vi "PAX_Read.vi"(8 "error in (no error)":errorcluster {"code" format="%.0x"}, 11 "VISA in":refnum<visa-resource-name> caption="instrument handle") -> (0 "error out":errorcluster {"code" format="%.0x"}, 1 "DOP":dbl, 2 "Azimuth deg":dbl, 3 "VISAout":refnum<visa-resource-name> caption="instrument handle out", 4 "s1":dbl, 5 "Ellipticity deg":dbl caption="Ellipticity rad", 6 "s3":dbl, 7 "s2":dbl)   [LabVIEW 2018]
panel:
  out "Total Power":dbl
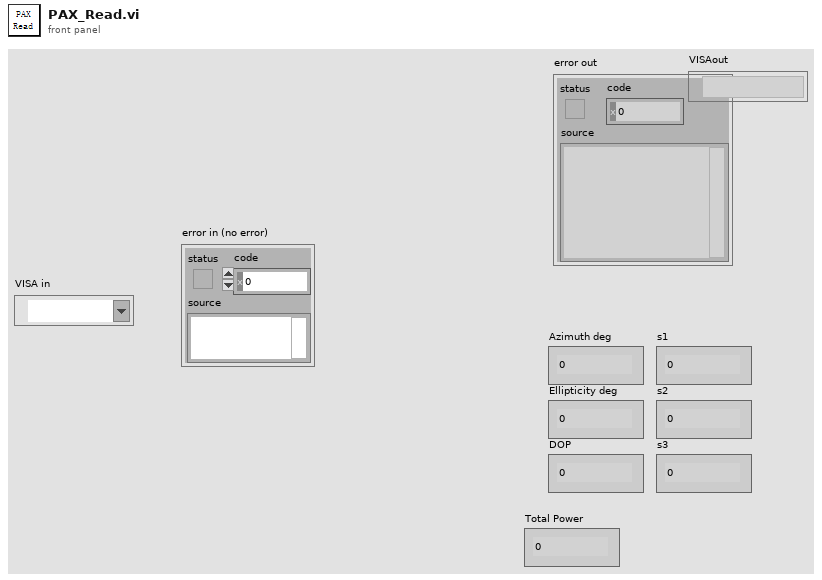
[diagram p1: front panel]
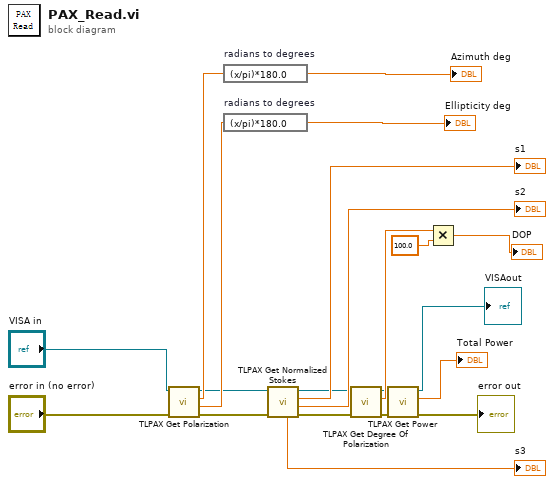
[diagram p0: block diagram]
diagram:
  n1 = call <instrlib>:"TLPAX Get Polarization.vi"("error in (no error)"="error in (no error)", "instrument handle"="VISA in") -> ("error out"=w6:errorcluster, "Ellipticity rad"=w18:dbl, "Azimuth rad"=w19:dbl, "instrument handle out"=w7:refnum<visa-resource-name>)  [unwired: 6 in]
  n2 = expression code="(x/pi)*180.0" "radians to degrees"(w19) -> (→"Azimuth deg":dbl)
  n3 = expression code="(x/pi)*180.0" "radians to degrees"(w18) -> (→"Ellipticity deg":dbl)
  n4 = call <instrlib>:"TLPAX Get Normalized Stokes.vi"("error in (no error)"=w6, "instrument handle"=w7) -> ("error out"=w11:errorcluster, "s2"=→"s2":dbl, "s1"=→"s1":dbl, "instrument handle out"=w10:refnum<visa-resource-name>, "s3"=→"s3":dbl)  [unwired: 5 in]
  n5 = call <instrlib>:"TLPAX Get Degree Of Polarization.vi"("error in (no error)"=w11, "instrument handle"=w10) -> ("error out"=w9:errorcluster, "DOP"=w14:dbl, "instrument handle out"=w8:refnum<visa-resource-name>)  [unwired: 5 in, 2 out]
  n6 = call <instrlib>:"TLPAX Get Power.vi"("error in (no error)"=w9, "instrument handle"=w8) -> ("error out"=→"error out":errorcluster, "Total Power"=→"Total Power":dbl, "instrument handle out"=→"VISAout":refnum<visa-resource-name>)  [unwired: 5 in, 2 out]
  n7 = Multiply(x=w14, y=100.0) -> (x*y=→"DOP":dbl)
